vi "2022teikyou.myrio-01.vi"() -> ()   [LabVIEW 2017]
uses:
  LabVIEW Data/myRIO_2021_ARC/RT VIs/RT Global.vi
panel:
  in  "Error/Flow In 2":errorcluster
  in  "stop 2":bool
  out "Error/Flow Out 2":errorcluster
  out "´¹g@E":i32
  out "´¹g@¶":i32
  out "Error/Flow Out":errorcluster
  in  "Error/Flow In":errorcluster
  out "—Îx":sgl
  out "Ôx":sgl
  in  "stop":bool
  out "Image Out":T1(plugin-control)
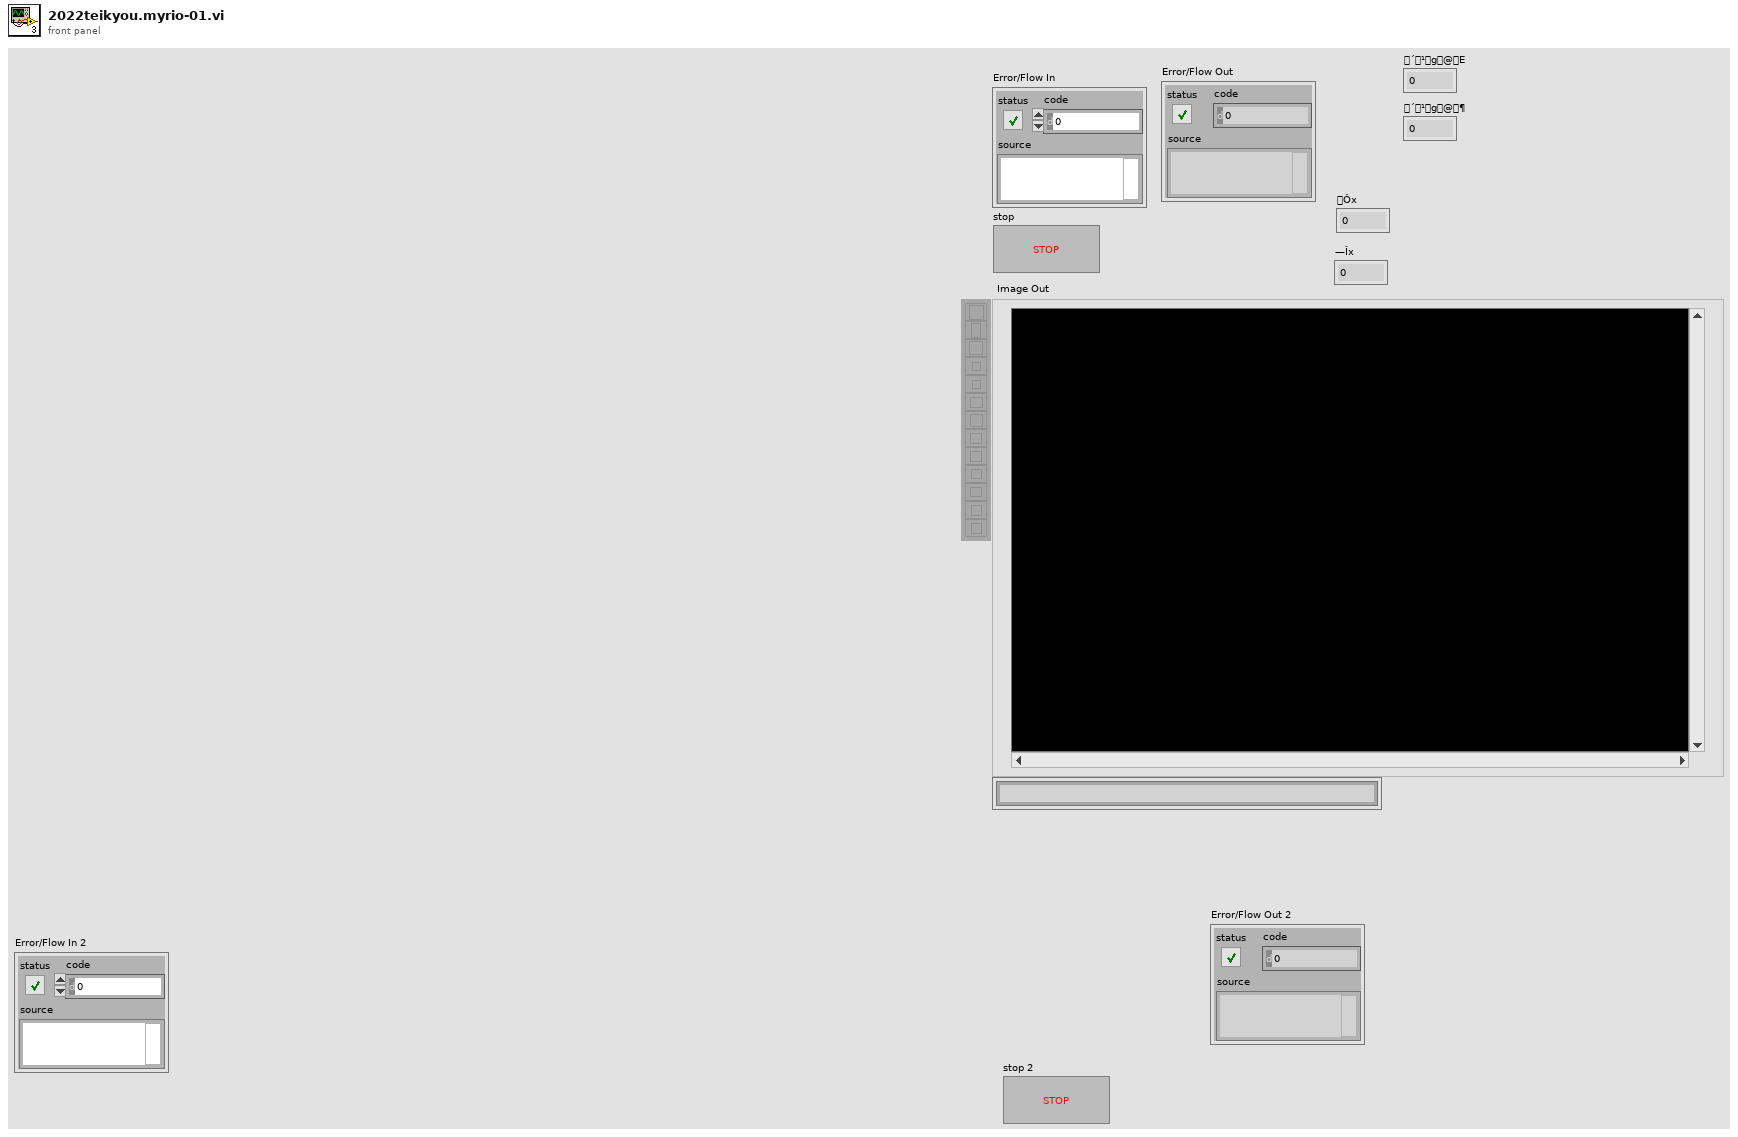
[diagram p1: front panel]
types:
  T1 = typedef "IMAQ Image.ctl" = refnum<image>
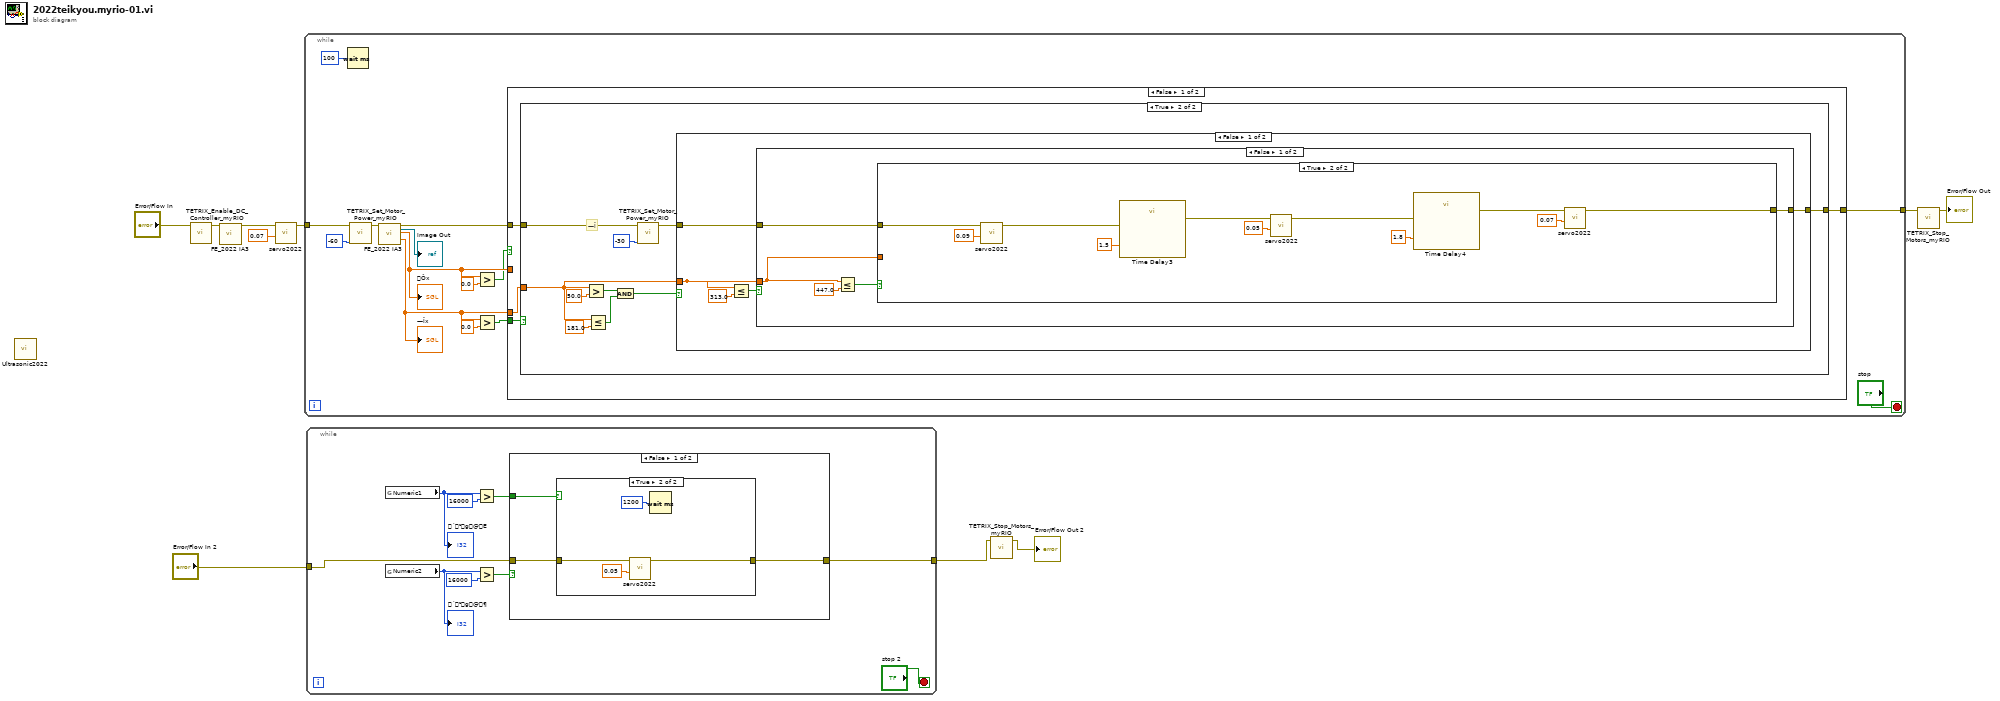
[diagram p0: block diagram]
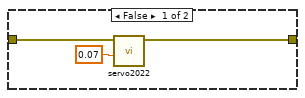
[diagram p2: hidden frame]
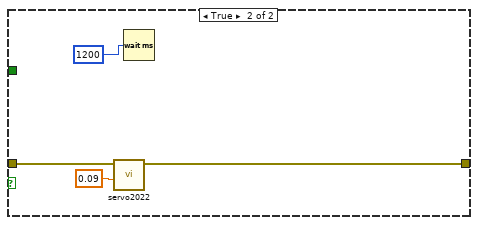
[diagram p3: hidden frame]
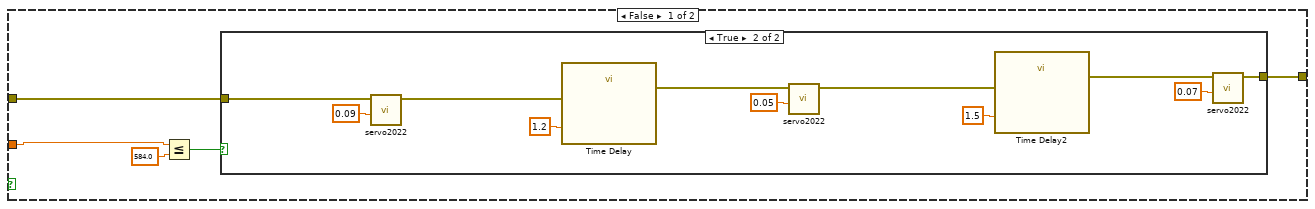
[diagram p5: hidden frame]
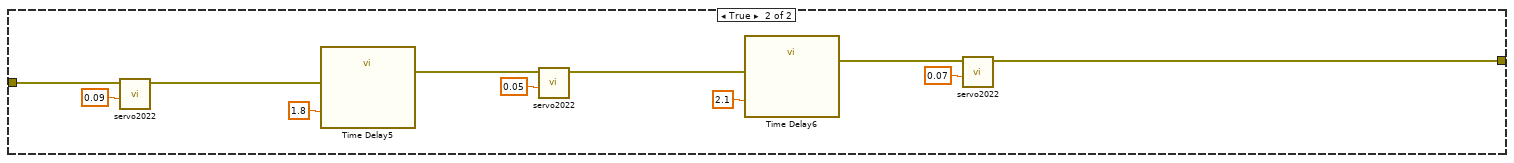
[diagram p7: hidden frame]
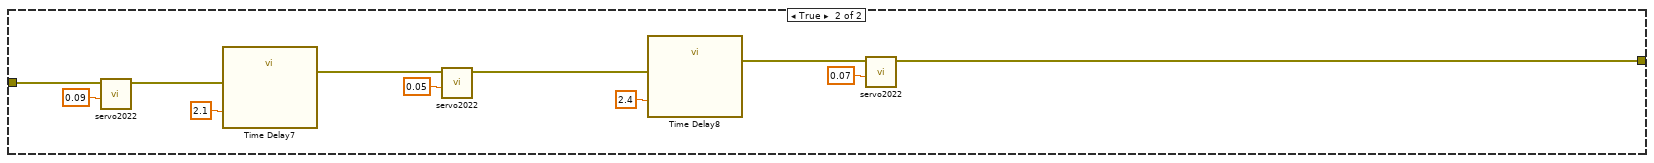
[diagram p8: hidden frame]
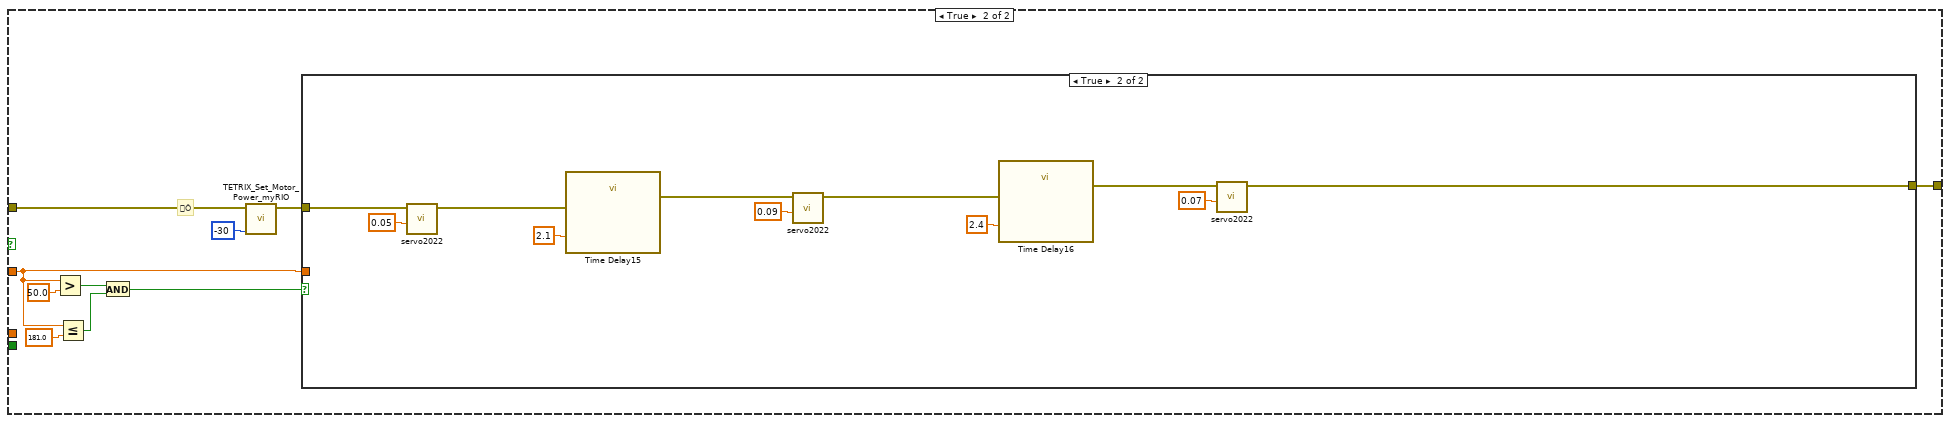
[diagram p9: hidden frame]
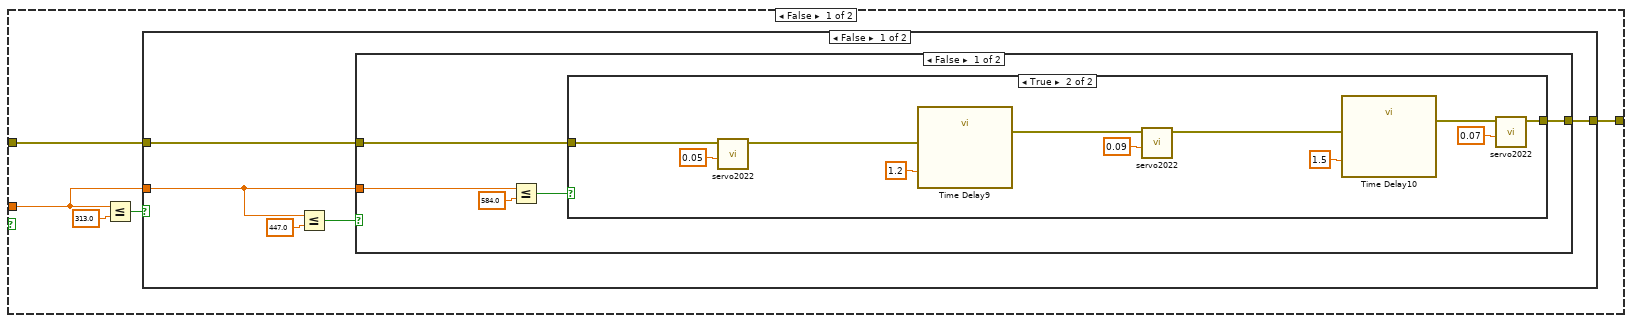
[diagram p10: hidden frame]
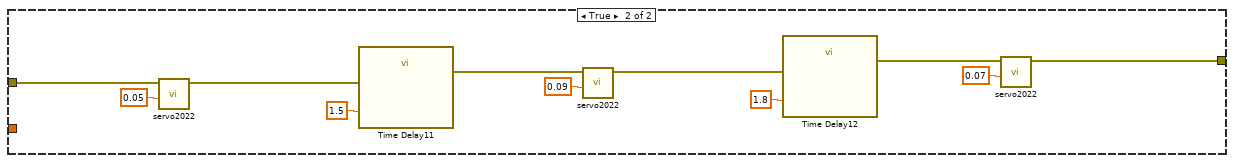
[diagram p12: hidden frame]
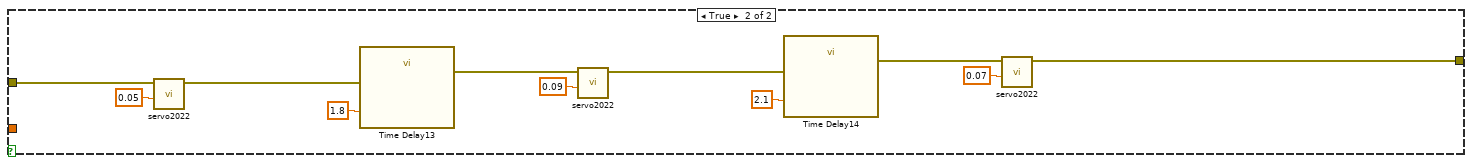
[diagram p13: hidden frame]
diagram:
  n1 = call "Ultrasonic2022.vi"() -> ()  [unwired: 10 in, 2 out]
  n2 = call <vilib>:"TETRIX_Enable_DC_Controller_myRIO.vi"("Error/Flow In"="Error/Flow In") -> ("Error/Flow Out"=w4:errorcluster)  [unwired: 6 in]
  n3 = call "FE_2022 IA3.vi"("error in"=w4) -> ("error out"=w7:errorcluster)  [unwired: 13 in, 5 out]
  n4 = call "servo2022.vi"("Duty Cycle"=0.07, "error out 2"=w7) -> ("error out"=w6:errorcluster)  [unwired: 9 in]
  n5 = while {
    tunnel: w6 -> [w24]
    tunnel: [w20] -> w9
    stop <- "stop" stop-if-true
    n6 = Wait (ms)(milliseconds to wait=u32 100) -> ()  [unwired: 1 out]
    n7 = call <vilib>:"TETRIX_Set_Motor_Power_myRIO.vi"("Power (-100 to 100)  0 = Coast Stop  125 = Brake Stop"=i8 -60, "Error/Flow In"=w24) -> ("Error/Flow Out"=w23:errorcluster)  [unwired: 5 in]
    n8 = call "FE_2022 IA3.vi"("error in"=w23) -> ("error out"=w22:errorcluster, "Image Out"=→"Image Out":T1, "Ôx"=w15:sgl, "—Îx"=w13:sgl)  [unwired: 13 in, 2 out]
    "—Îx" <- w13
    "Ôx" <- w15
    n9 = Greater?(x=w15, y=sgl 0.0) -> (0:w12:bool)
    n10 = Greater?(x=w13, y=sgl 0.0) -> (0:w11:bool)
    n11 = case shown="False" w12 {
      tunnel: w22 -> [w28 w102]
      tunnel: [w27 w105] -> w20
      tunnel: w13 -> [w26 _]
      tunnel: w15 -> [_ w103]
      tunnel: w11 -> [w25 _]
      frame False {
        n12 = case shown="True" w25 {
          tunnel: w28 -> [w29 w32]
          tunnel: [w29 w39] -> w27
          tunnel: w26 -> [_ w35]
          frame False {
          }
          frame True {
            # "—Î"
            n13 = Greater?(x=w35, y=sgl 50.0) -> (0:w38:bool)
            n14 = Less Or Equal?(x=w35, y=sgl 181.0) -> (x <= y?=w37:bool)
            n15 = And(x=w38, y=w37) -> (x .and. y?=w36:bool)
            n16 = call <vilib>:"TETRIX_Set_Motor_Power_myRIO.vi"("Power (-100 to 100)  0 = Coast Stop  125 = Brake Stop"=i8 -30, "Error/Flow In"=w32) -> ("Error/Flow Out"=w31:errorcluster)  [unwired: 5 in]
            n17 = case shown="False" w36 {
              tunnel: w31 -> [w44 w89]
              tunnel: [w43 w90] -> w39
              tunnel: w35 -> [w41 _]
              frame False {
                n18 = Less Or Equal?(x=w41, y=sgl 313.0) -> (x <= y?=w42:bool)
                n19 = case shown="False" w42 {
                  tunnel: w44 -> [w49 w78]
                  tunnel: [w48 w79] -> w43
                  tunnel: w41 -> [w46 _]
                  frame False {
                    n20 = Less Or Equal?(x=w46, y=sgl 447.0) -> (x <= y?=w47:bool)
                    n21 = case shown="True" w47 {
                      tunnel: w49 -> [w54 w69]
                      tunnel: [w53 w68] -> w48
                      tunnel: w46 -> [w52 _]
                      frame False {
                        n22 = Less Or Equal?(x=w52, y=sgl 584.0) -> (x <= y?=w51:bool)
                        n23 = case shown="True" w51 {
                          tunnel: w54 -> [w55 w57]
                          tunnel: [w55 w56] -> w53
                          frame False {
                          }
                          frame True {
                            n24 = call "servo2022.vi"("Duty Cycle"=0.09, "error out 2"=w57) -> ("error out"=w66:errorcluster)  [unwired: 9 in]
                            n25 = call "Time Delay"("error in (no error)"=w66, "Delay Time (s)"=1.2) -> ("error out"=w61:errorcluster)  [unwired: 9 in]
                            n26 = call "servo2022.vi"("Duty Cycle"=0.05, "error out 2"=w61) -> ("error out"=w62:errorcluster)  [unwired: 9 in]
                            n27 = call "Time Delay2"("error in (no error)"=w62, "Delay Time (s)"=1.5) -> ("error out"=w58:errorcluster)  [unwired: 9 in]
                            n28 = call "servo2022.vi"("Duty Cycle"=0.07, "error out 2"=w58) -> ("error out"=w56:errorcluster)  [unwired: 9 in]
                          }
                        }
                      }
                      frame True {
                        n29 = call "servo2022.vi"("Duty Cycle"=0.09, "error out 2"=w69) -> ("error out"=w77:errorcluster)  [unwired: 9 in]
                        n30 = call "Time Delay3"("error in (no error)"=w77, "Delay Time (s)"=1.5) -> ("error out"=w72:errorcluster)  [unwired: 9 in]
                        n31 = call "servo2022.vi"("Duty Cycle"=0.05, "error out 2"=w72) -> ("error out"=w73:errorcluster)  [unwired: 9 in]
                        n32 = call "Time Delay4"("error in (no error)"=w73, "Delay Time (s)"=1.8) -> ("error out"=w70:errorcluster)  [unwired: 9 in]
                        n33 = call "servo2022.vi"("Duty Cycle"=0.07, "error out 2"=w70) -> ("error out"=w68:errorcluster)  [unwired: 9 in]
                      }
                    }
                  }
                  frame True {
                    n34 = call "servo2022.vi"("Duty Cycle"=0.09, "error out 2"=w78) -> ("error out"=w88:errorcluster)  [unwired: 9 in]
                    n35 = call "Time Delay5"("error in (no error)"=w88, "Delay Time (s)"=1.8) -> ("error out"=w83:errorcluster)  [unwired: 9 in]
                    n36 = call "servo2022.vi"("Duty Cycle"=0.05, "error out 2"=w83) -> ("error out"=w84:errorcluster)  [unwired: 9 in]
                    n37 = call "Time Delay6"("error in (no error)"=w84, "Delay Time (s)"=2.1) -> ("error out"=w80:errorcluster)  [unwired: 9 in]
                    n38 = call "servo2022.vi"("Duty Cycle"=0.07, "error out 2"=w80) -> ("error out"=w79:errorcluster)  [unwired: 9 in]
                  }
                }
              }
              frame True {
                n39 = call "servo2022.vi"("Duty Cycle"=0.09, "error out 2"=w89) -> ("error out"=w99:errorcluster)  [unwired: 9 in]
                n40 = call "Time Delay7"("error in (no error)"=w99, "Delay Time (s)"=2.1) -> ("error out"=w94:errorcluster)  [unwired: 9 in]
                n41 = call "servo2022.vi"("Duty Cycle"=0.05, "error out 2"=w94) -> ("error out"=w95:errorcluster)  [unwired: 9 in]
                n42 = call "Time Delay8"("error in (no error)"=w95, "Delay Time (s)"=2.4) -> ("error out"=w91:errorcluster)  [unwired: 9 in]
                n43 = call "servo2022.vi"("Duty Cycle"=0.07, "error out 2"=w91) -> ("error out"=w90:errorcluster)  [unwired: 9 in]
              }
            }
          }
        }
      }
      frame True {
        # "Ô"
        n44 = Greater?(x=w103, y=sgl 50.0) -> (0:w108:bool)
        n45 = Less Or Equal?(x=w103, y=sgl 181.0) -> (x <= y?=w107:bool)
        n46 = And(x=w108, y=w107) -> (x .and. y?=w106:bool)
        n47 = call <vilib>:"TETRIX_Set_Motor_Power_myRIO.vi"("Power (-100 to 100)  0 = Coast Stop  125 = Brake Stop"=i8 -30, "Error/Flow In"=w102) -> ("Error/Flow Out"=w101:errorcluster)  [unwired: 5 in]
        n48 = case shown="True" w106 {
          tunnel: w101 -> [w113 w160]
          tunnel: [w112 w159] -> w105
          tunnel: w103 -> [w110 _]
          frame False {
            n49 = Less Or Equal?(x=w110, y=sgl 313.0) -> (x <= y?=w114:bool)
            n50 = case shown="False" w114 {
              tunnel: w113 -> [w117 w148]
              tunnel: [w118 w149] -> w112
              tunnel: w110 -> [w115 _]
              frame False {
                n51 = Less Or Equal?(x=w115, y=sgl 447.0) -> (x <= y?=w119:bool)
                n52 = case shown="False" w119 {
                  tunnel: [w121 w138] -> w118
                  tunnel: w117 -> [w120 w137]
                  tunnel: w115 -> [w124 _]
                  frame False {
                    n53 = Less Or Equal?(x=w124, y=sgl 584.0) -> (x <= y?=w122:bool)
                    n54 = case shown="True" w122 {
                      tunnel: [w125 w126] -> w121
                      tunnel: w120 -> [w125 w127]
                      frame False {
                      }
                      frame True {
                        n55 = call "servo2022.vi"("Duty Cycle"=0.05, "error out 2"=w127) -> ("error out"=w136:errorcluster)  [unwired: 9 in]
                        n56 = call "Time Delay9"("error in (no error)"=w136, "Delay Time (s)"=1.2) -> ("error out"=w131:errorcluster)  [unwired: 9 in]
                        n57 = call "servo2022.vi"("Duty Cycle"=0.09, "error out 2"=w131) -> ("error out"=w132:errorcluster)  [unwired: 9 in]
                        n58 = call "Time Delay10"("error in (no error)"=w132, "Delay Time (s)"=1.5) -> ("error out"=w128:errorcluster)  [unwired: 9 in]
                        n59 = call "servo2022.vi"("Duty Cycle"=0.07, "error out 2"=w128) -> ("error out"=w126:errorcluster)  [unwired: 9 in]
                      }
                    }
                  }
                  frame True {
                    n60 = call "servo2022.vi"("Duty Cycle"=0.05, "error out 2"=w137) -> ("error out"=w147:errorcluster)  [unwired: 9 in]
                    n61 = call "Time Delay11"("error in (no error)"=w147, "Delay Time (s)"=1.5) -> ("error out"=w142:errorcluster)  [unwired: 9 in]
                    n62 = call "servo2022.vi"("Duty Cycle"=0.09, "error out 2"=w142) -> ("error out"=w143:errorcluster)  [unwired: 9 in]
                    n63 = call "Time Delay12"("error in (no error)"=w143, "Delay Time (s)"=1.8) -> ("error out"=w139:errorcluster)  [unwired: 9 in]
                    n64 = call "servo2022.vi"("Duty Cycle"=0.07, "error out 2"=w139) -> ("error out"=w138:errorcluster)  [unwired: 9 in]
                  }
                }
              }
              frame True {
                n65 = call "servo2022.vi"("Duty Cycle"=0.05, "error out 2"=w148) -> ("error out"=w158:errorcluster)  [unwired: 9 in]
                n66 = call "Time Delay13"("error in (no error)"=w158, "Delay Time (s)"=1.8) -> ("error out"=w153:errorcluster)  [unwired: 9 in]
                n67 = call "servo2022.vi"("Duty Cycle"=0.09, "error out 2"=w153) -> ("error out"=w154:errorcluster)  [unwired: 9 in]
                n68 = call "Time Delay14"("error in (no error)"=w154, "Delay Time (s)"=2.1) -> ("error out"=w150:errorcluster)  [unwired: 9 in]
                n69 = call "servo2022.vi"("Duty Cycle"=0.07, "error out 2"=w150) -> ("error out"=w149:errorcluster)  [unwired: 9 in]
              }
            }
          }
          frame True {
            n70 = call "servo2022.vi"("Duty Cycle"=0.05, "error out 2"=w160) -> ("error out"=w169:errorcluster)  [unwired: 9 in]
            n71 = call "Time Delay15"("error in (no error)"=w169, "Delay Time (s)"=2.1) -> ("error out"=w164:errorcluster)  [unwired: 9 in]
            n72 = call "servo2022.vi"("Duty Cycle"=0.09, "error out 2"=w164) -> ("error out"=w165:errorcluster)  [unwired: 9 in]
            n73 = call "Time Delay16"("error in (no error)"=w165, "Delay Time (s)"=2.4) -> ("error out"=w161:errorcluster)  [unwired: 9 in]
            n74 = call "servo2022.vi"("Duty Cycle"=0.07, "error out 2"=w161) -> ("error out"=w159:errorcluster)  [unwired: 9 in]
          }
        }
      }
    }
  }
  n75 = while {
    tunnel: [w173] -> w2
    tunnel: "Error/Flow In 2" -> [w171]
    stop <- "stop 2" stop-if-true
    n76 = global read "RT Global.vi" "Numeric1"() -> (w170:i32)
    "´¹g@E" <- w170
    n77 = global read "RT Global.vi" "Numeric2"() -> (w178:i32)
    "´¹g@¶" <- w178
    n78 = Greater?(x=w170, y=u32 16000) -> (0:w175:bool)
    n79 = Greater?(x=w178, y=16000) -> (0:w174:bool)
    n80 = case shown="False" w174 {
      tunnel: w171 -> [w180 w190]
      tunnel: [w181 w189] -> w173
      tunnel: w175 -> [w179 _]
      frame False {
        n81 = case shown="True" w179 {
          tunnel: w180 -> [w184 w187]
          tunnel: [w183 w186] -> w181
          frame False {
            n82 = call "servo2022.vi"("Duty Cycle"=0.07, "error out 2"=w184) -> ("error out"=w183:errorcluster)  [unwired: 9 in]
          }
          frame True {
            n83 = call "servo2022.vi"("Duty Cycle"=0.05, "error out 2"=w187) -> ("error out"=w186:errorcluster)  [unwired: 9 in]
            n84 = Wait (ms)(milliseconds to wait=u32 1200) -> ()  [unwired: 1 out]
          }
        }
      }
      frame True {
        n85 = call "servo2022.vi"("Duty Cycle"=0.09, "error out 2"=w190) -> ("error out"=w189:errorcluster)  [unwired: 9 in]
        n86 = Wait (ms)(milliseconds to wait=u32 1200) -> ()  [unwired: 1 out]
      }
    }
  }
  n87 = call <vilib>:"TETRIX_Stop_Motors_myRIO.vi"("Error/Flow In"=w2) -> ("Error/Flow Out"=→"Error/Flow Out 2":errorcluster)  [unwired: 6 in]
  n88 = call <vilib>:"TETRIX_Stop_Motors_myRIO.vi"("Error/Flow In"=w9) -> ("Error/Flow Out"=→"Error/Flow Out":errorcluster)  [unwired: 6 in]
